vi "IPI_Cal_Radio.vi"(0 "X plus":string, 1 "Y plus":string, 2 "U plus":string, 3 "X MM":string, 4 "Y MM":string, 5 "U MM":string) -> (14 "X raido":string, 16 "Y raido":string, 18 "U raido":string)   [LabVIEW 2015]
panel:
  out "F-格式字符串":string[](array[string])
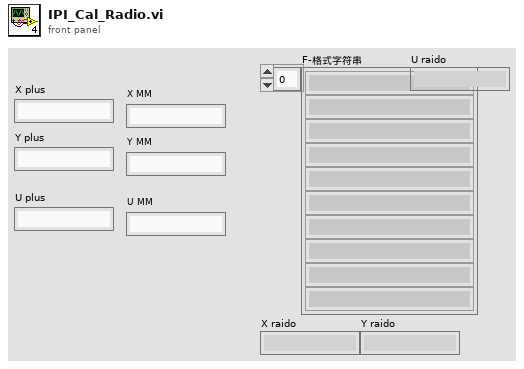
[diagram p1: front panel]
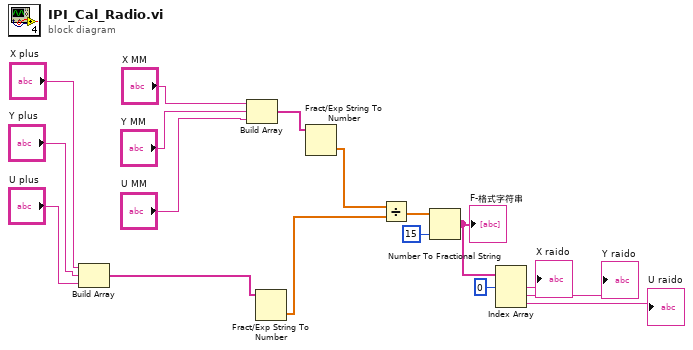
[diagram p0: block diagram]
diagram:
  n1 = Build Array("X plus", "Y plus", "U plus") -> (w10:string[])
  n2 = Build Array("X MM", "Y MM", "U MM") -> (w11:string[])
  n3 = Fract/Exp String To Number(string=w10) -> (number=w8:dbl[])  [unwired: 3 in, 1 out]
  n4 = Fract/Exp String To Number(string=w11) -> (number=w9:dbl[])  [unwired: 3 in, 1 out]
  n5 = Divide(x=w9, y=w8) -> (x/y=w7:dbl[])
  n6 = Number To Fractional String(number=w7, precision (6)=i16 15 ("精度(6)")) -> (F-format string=w5:string[])  [unwired: 2 in]
  "F-格式字符串" <- w5
  n7 = Index Array(array=w5, index #1=0 ("索引")) -> (element #1=→"X raido":string, element #2=→"Y raido":string, element #3=→"U raido":string)  [unwired: 2 in]
